vi "Save TestStand ResultList From Column to Excel.vi"(0 "Sequence Context":T1, 1 "Headers Path":path, 2 "report file path":path, 3 "start cell":cluster{"row":i32, "column":i32}, 4 "Column Name":string, 5 "error in (no error)":errorcluster, 7 "WriteTheHeaders":bool) -> (17 "next cell":cluster{"row":i32, "column":i32}, 19 "error out":errorcluster)   [LabVIEW 2015]
doc: "This vi will search the array of column names for Column Name\nand save an array of results starting at the point where Column Name is found\nBe sure to copy the name of the first Step with a result to the Column Name input"
uses:
  <vilib>/addons/TestStand/_TSLegacy.llb/LabVIEW Test - Sequence Context.ctl
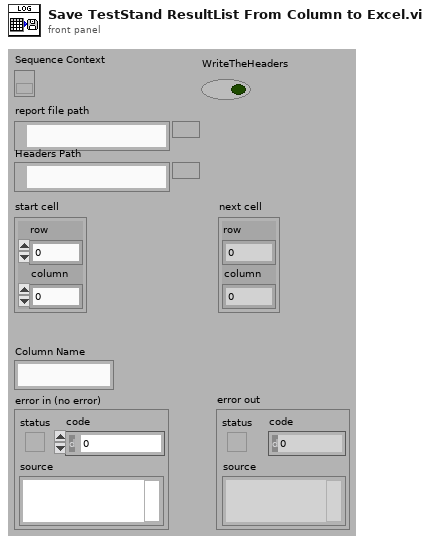
[diagram p1: front panel]
types:
  T1 = typedef "LabVIEW Test - Sequence Context.ctl" = refnum<k7>
  T2 = typedef "Test Result.ctl" = cluster{"StepName":string, "Status":bool, "Data":string, "Limits":variant}
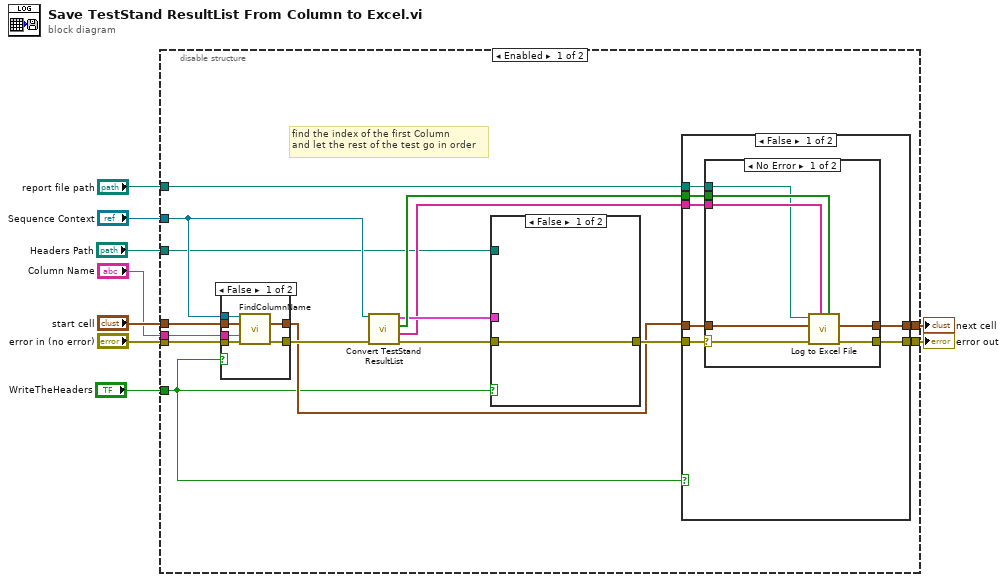
[diagram p0: block diagram]
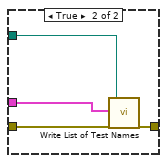
[diagram p5: hidden frame]
diagram:
  n1 = disable-structure shown="Enabled" {
    disable-tunnel: [w24 _] -> w9
    disable-tunnel: "report file path" -> [w23 _]
    disable-tunnel: [w22 _] -> w7
    disable-tunnel: "Sequence Context" -> [w21 _]
    disable-tunnel: "error in (no error)" -> [w20 _]
    disable-tunnel: "start cell" -> [w18 _]
    disable-tunnel: "Column Name" -> [w13 _]
    disable-tunnel: "Headers Path" -> [w11 _]
    disable-tunnel: "WriteTheHeaders" -> [w10 _]
    frame Enabled {
      # "find the index of the first Column\nand let the rest of the test go in order"
      n2 = case shown="False" w10 {
        tunnel: w21 -> [w31 _]
        tunnel: w20 -> [w30 w32]
        tunnel: [w29 w32] -> w19
        tunnel: w18 -> [w28 w33]
        tunnel: [w27 w33] -> w14
        tunnel: w13 -> [w26 _]
        frame False {
          n3 = call "FindColumnName.vi"("Sequence Context"=w31, "start cell in"=w28, "Column Name"=w26, "error in (no error)"=w30) -> ("start cell out"=w27:cluster{"row":i32, "column":i32}, "error out"=w29:errorcluster)  [unwired: 10 in]
        }
        frame True {
        }
      }
      n4 = call "Convert TestStand ResultList.vi"("error in (no error)"=w19, "Sequence Context"=w21) -> ("error out"=w17:errorcluster, "data"=w12:string[], "status"=w25:bool[], "Results"=w15:T2[])  [unwired: 6 in]
      n5 = case shown="False" w10 {
        tunnel: w17 -> [w52 w56]
        tunnel: [w52 w55] -> w16
        tunnel: w15 -> [_ w54]
        tunnel: w11 -> [_ w53]
        frame False {
        }
        frame True {
          n6 = call "Write List of Test Names.vi"("Results"=w54, "error in (no error)"=w56, "file path (use dialog)"=w53) -> ("error out"=w55:errorcluster)  [unwired: 16 in]
        }
      }
      n7 = case shown="False" w10 {
        tunnel: w25 -> [w40 _]
        tunnel: [w39 w51] -> w24
        tunnel: w23 -> [w38 _]
        tunnel: [w37 w50] -> w22
        tunnel: w16 -> [w36 w51]
        tunnel: w14 -> [w35 w50]
        tunnel: w12 -> [w34 _]
        frame False {
          n8 = case shown="No Error" w36 {
            selector: w36 -> [w41 w49]
            tunnel: w40 -> [w47 _]
            tunnel: w34 -> [w46 _]
            tunnel: [w45 w49] -> w39
            tunnel: w38 -> [w44 _]
            tunnel: w35 -> [w42 w48]
            tunnel: [w43 w48] -> w37
            frame No Error {
              n9 = call "Log to Excel File.vi"("status"=w47, "data"=w46, "error in"=w41, "start cell"=w42, "report file path"=w44) -> ("error out"=w45:errorcluster, "next cell"=w43:cluster{"row":i32, "column":i32})  [unwired: 5 in]
            }
            frame Error {
            }
          }
        }
        frame True {
        }
      }
    }
    frame Disabled {
    }
  }
  "error out" <- w9
  "next cell" <- w7
